vi "Get All VI Data.vi"(8 "error in (no error)":errorcluster, 11 "Path":path) -> (0 "error out":errorcluster, 3 "Item Data":refnum<class "Item.lvclass">[](array[class]))   [LabVIEW 2020, in "VI Properties Editor.lvlib"]
doc: "Gets all VI data from the source of VIs located at <B>Path</B>."
uses:
  VI Properties Editor.lvlib
  Classes/Item/Item.lvclass
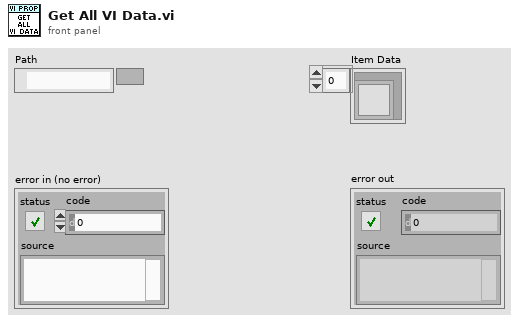
[diagram p1: front panel]
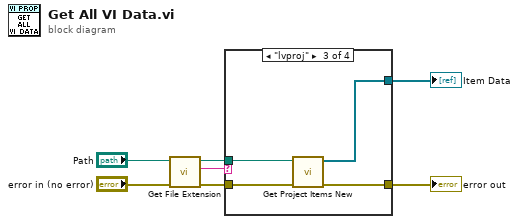
[diagram p0: block diagram]
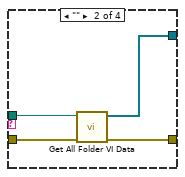
[diagram p3: hidden frame]
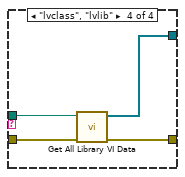
[diagram p4: hidden frame]
diagram:
  n1 = call <vilib>:"Get File Extension.vi"("error in (no error)"="error in (no error)", "file"="Path") -> ("error out"=w3:errorcluster, "lowercase file extension"=w5:string, "dup file"=w4:path)  [unwired: 5 in, 2 out]
  n2 = case shown="\"lvproj\"" w5 {
    tunnel: w4 -> [_ w11 w15 w19]
    tunnel: w3 -> [w8 w12 w16 w20]
    tunnel: [w8 w10 w14 w18] -> w2
    tunnel: [_ w9 w13 w17] -> w1
    frame Default {
    }
    frame "" {
      n3 = call "Get All Folder VI Data.vi"("error in (no error)"=w12, "Folder Path"=w11) -> ("error out"=w10:errorcluster, "Item Data"=w9:refnum<class "Item.lvclass">[])  [unwired: 8 in]
    }
    frame "lvproj" {
      n4 = call "Get Project Items New.vi"("error in (no error)"=w16, "Path"=w15) -> ("error out"=w14:errorcluster, "Items Data"=w13:refnum<class "Item.lvclass">[])  [unwired: 8 in]
    }
    frame "lvclass", "lvlib" {
      n5 = call "Get All Library VI Data.vi"("error in"=w20, "Lvlib Path"=w19) -> ("error out"=w18:errorcluster, "Item Data"=w17:refnum<class "Item.lvclass">[])  [unwired: 8 in]
    }
  }
  "error out" <- w2
  "Item Data" <- w1
